vi "CloseHandle.vi"(4 "error in (no error)":errorcluster, 7 "hObject (NULL)":i32 format="%.0x") -> (0 "error out":errorcluster)   [LabVIEW 2011]
uses:
  KERNEL32.DLL
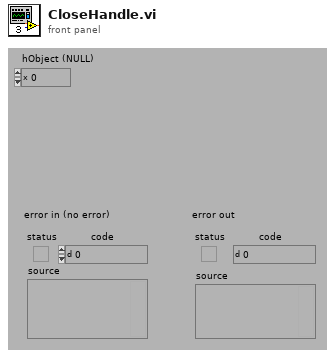
[diagram p1: front panel]
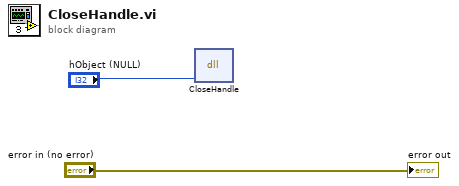
[diagram p0: block diagram]
diagram:
  n1 = dll-call lib="KERNEL32.DLL" fn="CloseHandle" label="CloseHandle()"("hObject"="hObject (NULL)") -> ()  [unwired: 4 in, 3 out]
  "error out" <- "error in (no error)"
